vi "Teleop.vi"(10 "Match Info":T1={"Autonomous Elapsed Seconds"=0.0, "TeleOp Elapsed Seconds"=0.0, "Disabled Elapsed Seconds"=0.0, "Visited Autonomous"=FALSE, "Visited TeleOp"=FALSE, "Visited Disabled"=FALSE, "Autonomous Settings"={"Autonomous Style"=enum."Independent", "VI Refnum"=refnum}}, 11 "Call Context":T2) -> ()   [LabVIEW 2012]
doc: "This VI is called for each TeleOp packet received from the DS where the robot is not disabled. It is often used to read from the joysticks and update I/O or to update setpoints for timed control loops. It should complete and return within 20 milliseconds or it may miss DS packets."
uses:
  <vilib>/Rock Robotics/WPI/DriverStation/WPI_DriverStationDerivedRobotMode.ctl
  <vilib>/Rock Robotics/WPI/DriverStation/WPI_DriverStationMatch Info.ctl
  Robot Global Data.vi
  <vilib>/Rock Robotics/WPI/Joystick/WPI_JoystickGetSetRefNum.vi
  <vilib>/Rock Robotics/WPI/RobotDrive/WPI_RobotDriveGetSetRefNum.vi
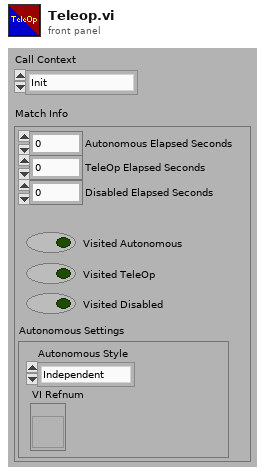
[diagram p1: front panel]
types:
  T1 = typedef "WPI_DriverStationMatch Info.ctl" = cluster{"Autonomous Elapsed Seconds":dbl, "TeleOp Elapsed Seconds":dbl, "Disabled Elapsed Seconds":dbl, "Visited Autonomous":bool, "Visited TeleOp":bool, "Visited Disabled":bool, "Autonomous Settings":cluster{"Autonomous Style":enum16{"Iterative", "Independent"}, "VI Refnum":refnum<vi>}}
  T2 = typedef "WPI_DriverStationDerivedRobotMode.ctl" = enum16{"Init", "Execute", "Stop"}
  T3 = typedef "WPI_JoystickDevRef.ctl" = cluster{"Device":T4}
  T4 = typedef "WPI_JoystickDeviceEnum.ctl" = enum16{"USB 1", "USB 2", "USB 3", "USB 4", "Kinect 1", "Kinect 2"}
  T5 = typedef "WPI_JoystickButtonState.ctl" = cluster{"Button 1":bool, "Button 2":bool, "Button 3":bool, "Button 4":bool, "Button 5":bool, "Button 6":bool, "Button 7":bool, "Button 8":bool, "Button 9":bool, "Button 10":bool, "Button 11":bool, "Button 12":bool}
  T6 = cluster{"axis 1 (x)":dbl, "axis 2 (y)":dbl, "axis 3 (throttle)":dbl, "axis 4":dbl, "axis 5":dbl, "axis 6":dbl}
  T7 = typedef "WPI_RobotDriveDevRef.ctl" = cluster{"DevStatus":errorcluster, "Motors[]":T8[], "Square Inputs":bool, "Max Output":dbl, "Isochronous":bool}
  T8 = typedef "WPI_MotorControlDeviceRef.ctl" = cluster{"DeviceStatus":errorcluster, "Type":enum16{"PWM", "CAN"}, "PWM":cluster{"Digital Module":T9, "PWM Channel":T10, "DeadBand":T11}, "CAN":cluster{"Device Number":u8, "Control Mode":T12, "Semaphore":T13, "Max Vout":dbl}, "Invert":bool, "TransformRef":T14, "InvTransformRef":T14}
  T9 = typedef "FPGA_TypedefDigitalModule.ctl" = enum16{"Digital Module 1", "Digital Module 2"}
  T10 = typedef "FPGA_DIOPWMChannel.ctl" = enum8{"PWM 1", "PWM 2", "PWM 3", "PWM 4", "PWM 5", "PWM 6", "PWM 7", "PWM 8", "PWM 9", "PWM 10", "Invalid"}
  T11 = typedef "WPI_PWMDeadband.ctl" = cluster{"Name":string, "maxPositivePwm":i32, "minPositivePwm":i32, "centerPwm":i32, "maxNegativePwm":i32, "minNegativePwm":i32, "angularRange":u16}
  T12 = typedef "WPI_CANJaguar_ControlMode.ctl" = enum8{"Percent VBus", "Current", "Speed", "Position", "Voltage"}
  T13 = typedef "Semaphore RefNum" = refnum<k1>
  T14 = typedef "WPI_PWMTransform_ConPane.ctl" = refnum<vi>
  T15 = enum16{"Off", "Close Pyramid 3pt", "Far Pyramid 3pt", "Feeder Shot"}
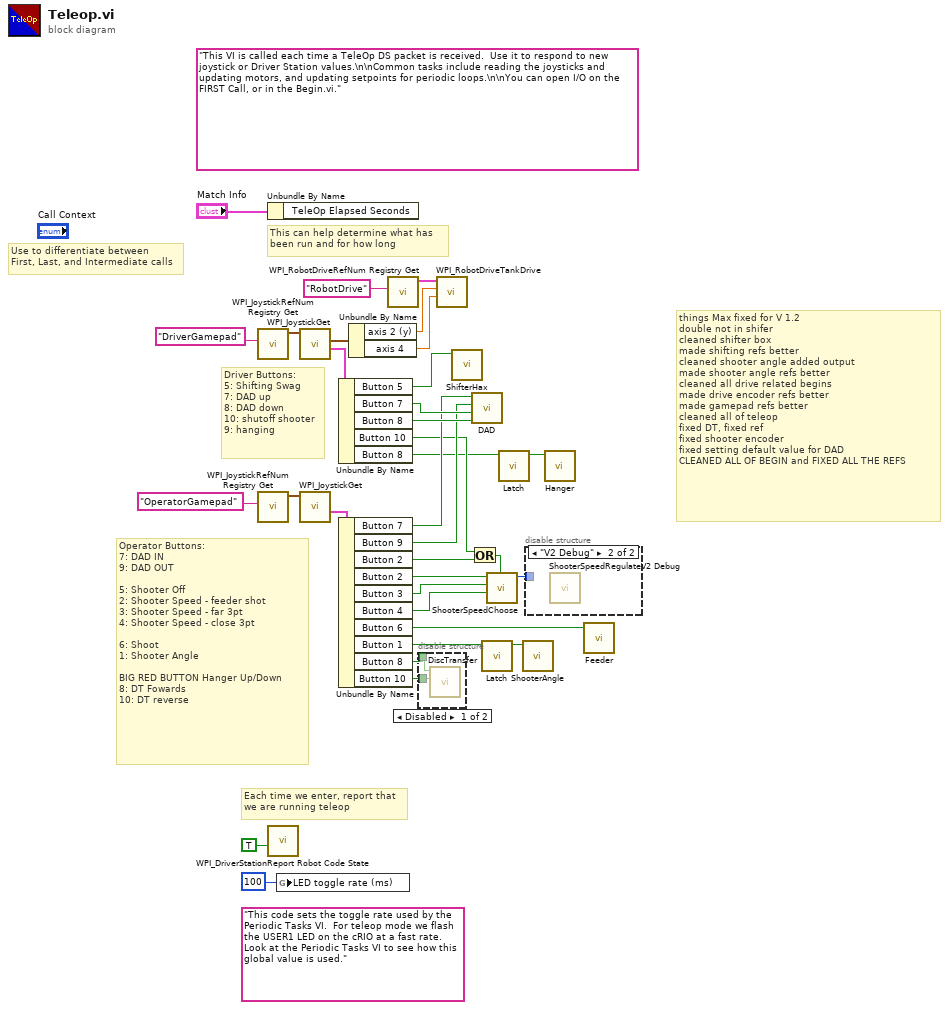
[diagram p0: block diagram]
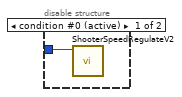
[diagram p3: hidden frame]
diagram:
  (unwired) "This code sets the toggle rate used by the Periodic Tasks VI.  For teleop mode we flash the USER1 LED on the cRIO at a fast rate.  Look at the Periodic Tasks VI to see how this global value is used."
  (unwired) "This VI is called each time a TeleOp DS packet is received.  Use it to respond to new joystick or Driver Station values.\n\nCommon tasks include reading the joysticks and updating motors, and updating setpoints for periodic loops.\n\nYou can open I/O on the FIRST Call, or in the Begin.vi."
  # "things Max fixed for V 1.2\ndouble not in shifer\ncleaned shifter box\nmade shifting refs better\ncleaned shooter angle added output\nmade shooter angle refs better\ncleaned all drive related begins\nmade drive encoder refs better\nmade gamepad refs better\ncleaned all of teleop\nfixed DT, fixed ref\nfixed shooter encoder\nfixed setting default value for DAD\nCLEANED ALL OF BEGIN and FIXED ALL THE REFS"
  # "Driver Buttons:\n5: Shifting Swag\n7: DAD up\n8: DAD down \n10: shutoff shooter\n9: hanging"
  # "Operator Buttons:\n7: DAD IN\n9: DAD OUT\n\n5: Shooter Off\n2: Shooter Speed - feeder shot\n3: Shooter Speed - far 3pt\n4: Shooter Speed - close 3pt\n\n6: Shoot\n1: Shooter Angle\n\nBIG RED BUTTON Hanger Up/Down\n8: DT Fowards\n10: DT reverse"
  # "Each time we enter, report that\nwe are running teleop"
  # "Use to differentiate between\nFirst, Last, and Intermediate calls"
  # "This can help determine what has\nbeen run and for how long"
  n1 = call <vilib>:"WPI_JoystickRefNum Registry Get.vi"("refnum name"="DriverGamepad") -> ("JoystickDevRef"=w31:T3)  [unwired: 1 in, 9 out]
  n2 = call <vilib>:"WPI_JoystickRefNum Registry Get.vi"("refnum name"="OperatorGamepad") -> ("JoystickDevRef"=w25:T3)  [unwired: 1 in, 9 out]
  n3 = Unbundle By Name("Match Info") -> ()  [unwired: 1 out]
  n4 = call <vilib>:"WPI_DriverStationReport Robot Code State.vi"("TeleOp"=TRUE ("Autonomous")) -> ()  [unwired: 10 in, 1 out]
  n5 = global write "Robot Global Data.vi" "LED toggle rate (ms)"(u32 100 ("LED ms toggle rate")) -> ()
  n6 = call <vilib>:"WPI_JoystickGet.vi"("JoystickDevRef"=w31) -> ("Buttons"=w26:T5, "Axes"=w28:T6)  [unwired: 1 in, 4 out]
  n7 = call <vilib>:"WPI_JoystickGet.vi"("JoystickDevRef"=w25) -> ("Buttons"=w24:T5)  [unwired: 1 in, 5 out]
  n8 = Unbundle By Name(w26) -> ("Button 5"=w21:bool, "Button 7"=w17:bool, "Button 8"=w16:bool, "Button 10"=w12:bool, "Button 8"=w9:bool)
  n9 = Unbundle By Name(w24) -> ("Button 7"=w15:bool, "Button 9"=w14:bool, "Button 2"=w13:bool, "Button 2"=w6:bool, "Button 3"=w5:bool, "Button 4"=w4:bool, "Button 6"=w11:bool, "Button 1"=w10:bool, "Button 8"=w8:bool, "Button 10"=w7:bool)
  n10 = Unbundle By Name(w28) -> ("axis 2 (y)"=w2:dbl, "axis 4"=w1:dbl)
  n11 = call <vilib>:"WPI_RobotDriveRefNum Registry Get.vi"("refnum name"="RobotDrive") -> ("RobotDriveDevRef"=w27:T7)  [unwired: 1 in, 9 out]
  n12 = disable-structure shown="Disabled" {
    disable-tunnel: w8 -> [w35 _]
    disable-tunnel: w7 -> [w34 _]
    frame Disabled {
      n13 = call "DiscTransfer.vi"("DT Backwards"=w34, "DT Foward"=w35) -> ()  [unwired: 10 in]
    }
    frame Enabled {
    }
  }
  n14 = call <vilib>:"WPI_RobotDriveTankDrive.vi"("Right axis value"=w1, "Left axis value"=w2, "RobotDriveDevRef"=w27) -> ()  [unwired: 6 in, 3 out]
  n15 = call "ShifterHax.vi"("Shift low?"=w21) -> ()  [unwired: 11 in]
  n16 = Or(x=w12, y=w13) -> (x .or. y?=w3:bool)
  n17 = call "DAD.vi"("BAD DOWN"=w16, "BAD UP"=w17, "BAD OUT"=w14, "BAD IN"=w15) -> ()  [unwired: 7 in, 1 out]
  n18 = call "Latch.vi"("Latch In"=w10) -> ("Latch Out"=w20:bool)  [unwired: 10 in]
  n19 = call "ShooterSpeedChoose.vi"("Shooter OFF"=w3, "Close 3pt Shot Button"=w4, "Far 3pt Shot Button"=w5, "Feedershot Button"=w6) -> ("Shooter Speed"=w23:T15)  [unwired: 7 in]
  n20 = call "Latch.vi"("Latch In"=w9) -> ("Latch Out"=w22:bool)  [unwired: 10 in]
  n21 = call "ShooterAngle.vi"("Shooter Angle Up?"=w20) -> ()  [unwired: 10 in, 1 out]
  n22 = disable-structure shown="\"V2 Debug\"" {
    disable-tunnel: w23 -> [w36 _]
    frame condition #0 (active) {
      n23 = call "ShooterSpeedRegulateV2.vi"("Shooter Speed"=w36) -> ()  [unwired: 13 in, 2 out]
    }
    frame condition #1 {
      n24 = call "ShooterSpeedRegulateV2 Debug.vi"() -> ()  [unwired: 14 in, 2 out]
    }
  }
  n25 = call "Hanger.vi"("Hanger Up"=w22) -> ()  [unwired: 10 in, 1 out]
  n26 = call "Feeder.vi"("SHOOT Button"=w11) -> ()  [unwired: 10 in, 1 out]
